vi "Data Dialog.vi"(8 "error in (no error)":errorcluster, 10 "channel name(s)":string[](array[string]), 11 "Data":dbl[][](array[numeric])) -> (0 "error out":errorcluster)   [LabVIEW 2020]
panel:
  out "XY Graph":cluster{"X":dbl[], "Y":dbl[]}[](graph)
  out "SP Data Pk2Pk":string[][](table)
  in  "OK Button":bool
  out "Res Data":dbl[][](graph)
  out "power":bool
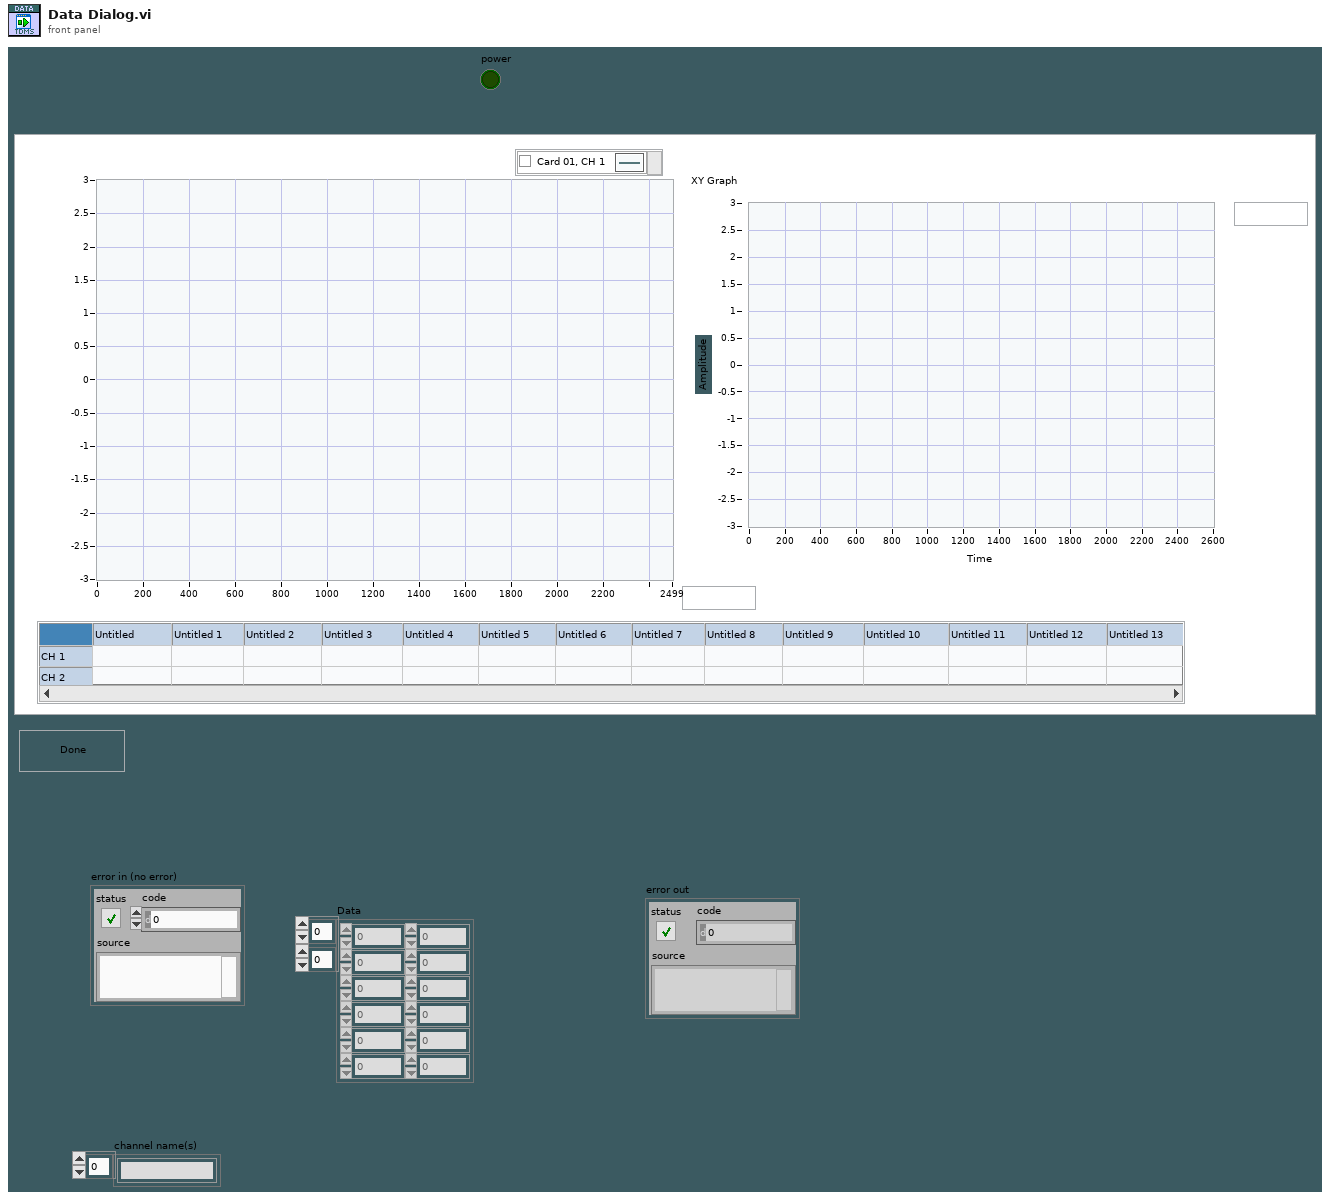
[diagram p1: front panel]
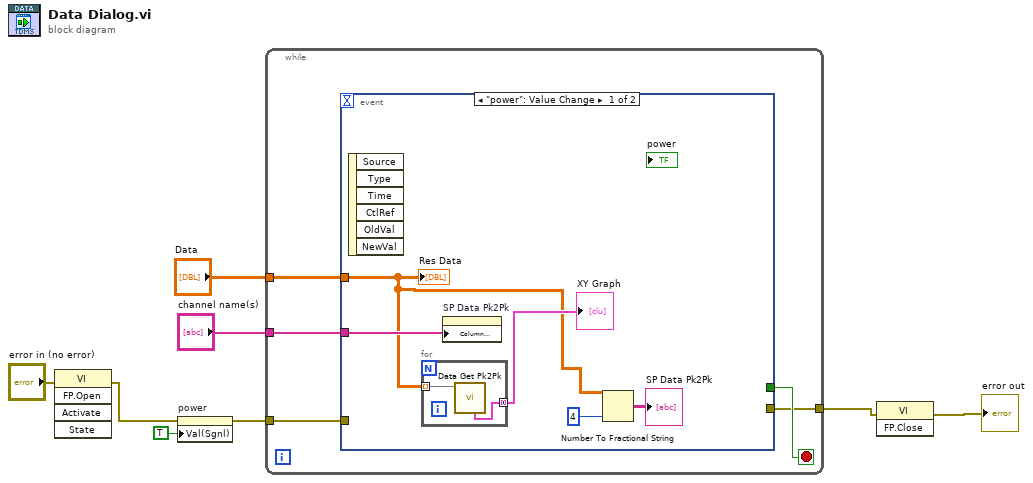
[diagram p0: block diagram]
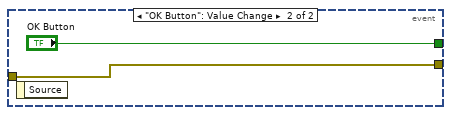
[diagram p2: hidden frame]
diagram:
  n1 = invoke class="VI" method="FP.Open"(error in="error in (no error)") -> (error out=w7:errorcluster)  [unwired: 4 in, 4 out]
  n2 = property on="power" class="Bool (strict)"(error in=w7, "Val(Sgnl)"=TRUE ("Value (Signaling)")) -> (error out=w6:errorcluster)  [unwired: 1 in, 1 out]
  n3 = while {
    tunnel: w6 -> [w11]
    tunnel: [w12] -> w5
    tunnel: "Data" -> [w10]
    tunnel: "channel name(s)" -> [w9]
    stop <- w13 stop-if-true
    n4 = event shown="[0] \"power\": Value Change" {
      selector: _ -> [_ _]
      dyn-events: _ -> [_ _]
      timeout: _ -> [_ _]
      tunnel: [_ "OK Button"] -> w13
      tunnel: [_ w21] -> w12
      tunnel: w11 -> [_ w21]
      tunnel: w10 -> [w14 _]
      tunnel: w9 -> [w16 _]
      event "power": Value Change {
        n5 = event-data() -> ()  [unwired: 1 in, 6 out]
        n6 = for {
          tunnel: w14 -> [w20] mode=indexing
          tunnel: [w19] -> w15 mode=concatenating
          n7 = call "Data Get Pk2Pk.vi"("Data"=w20) -> ("XY Graph"=w19:cluster{"X":dbl[], "Y":dbl[]}[])  [unwired: 10 in]
        }
        "XY Graph" <- w15
        n8 = property on="SP Data Pk2Pk" class="Tbl (strict)"("Column Headers[]"=w16) -> ()  [unwired: 2 in, 2 out]
        n9 = Number To Fractional String(number=w14, precision (6)=i16 4) -> (F-format string=→"SP Data Pk2Pk":string[][])  [unwired: 2 in]
        "Res Data" <- w14
      }
      event "OK Button": Value Change {
        n10 = event-data() -> ()  [unwired: 1 in, 1 out]
      }
    }
  }
  n11 = invoke class="VI" method="FP.Close"(error in=w5) -> (error out=→"error out":errorcluster)  [unwired: 2 in, 2 out]
